vi "main.vi"() -> ()   [LabVIEW 2018]
uses:
  <instrlib>/Tektronix AWG 5000 7000 Series/Public/Configure/Channel/Assign Output Waveform (From Waveform List).vi
  <instrlib>/Tektronix AWG 5000 7000 Series/Tektronix AWG 5000 7000 Series.lvlib
panel:
  in  "Wipe Names on execute":bool
  in  "Name 2":string
  in  "Amp 2":dbl
  in  "Amp 1":dbl
  in  "VISA name":refnum<visa-resource-name>
  in  "Frequency":dbl
  in  "Cant. Freq":dbl
  in  "Name":string
  in  "Max sample rate":dbl
  in  "Amplitude":dbl
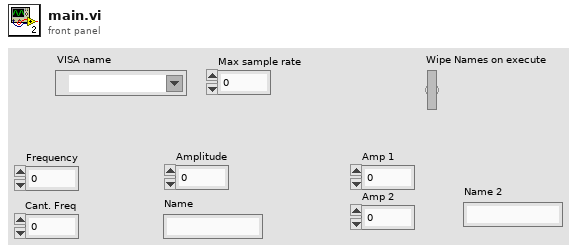
[diagram p1: front panel]
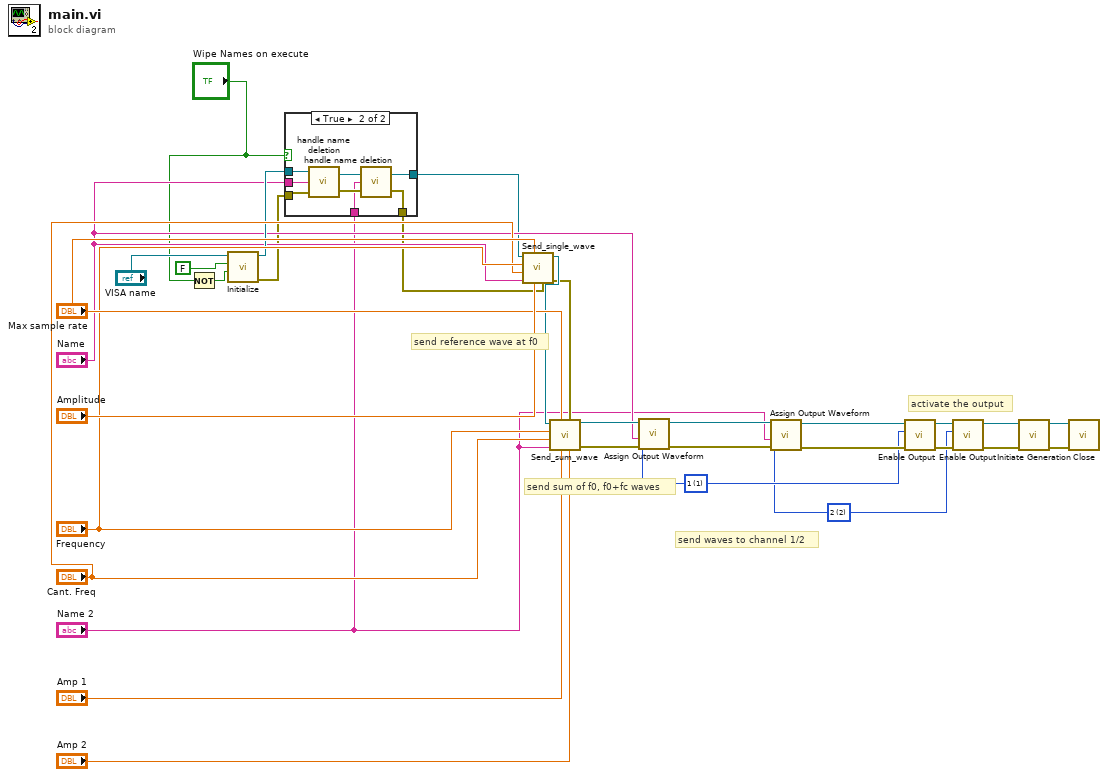
[diagram p0: block diagram]
diagram:
  w16 = u16 1 items=["1"=1, "2"=2, "3"=3, "4"=4] ("Channel Name (1)")
  w13 = u16 2 items=["1"=1, "2"=2, "3"=3, "4"=4] ("Channel Name (1)")
  # "activate the output"
  # "send waves to channel 1/2"
  # "send sum of f0, f0+fc waves"
  # "send reference wave at f0"
  n1 = Not(x="Wipe Names on execute") -> (.not. x?=w3:bool)
  n2 = call <instrlib>:"Initialize.vi"("Reset (False)"=w3, "ID Query (True)"=FALSE, "VISA resource name"="VISA name") -> ("error out"=w6:errorcluster, "VISA resource name out"=w8:refnum<visa-resource-name>)  [unwired: 7 in]
  n3 = case shown="True" "Wipe Names on execute" {
    tunnel: w8 -> [w33 w42]
    tunnel: "Name" -> [_ w41]
    tunnel: w6 -> [w34 w40]
    tunnel: [w33 w39] -> w5
    tunnel: [w34 w38] -> w4
    tunnel: "Name 2" -> [_ w35]
    frame False {
    }
    frame True {
      n4 = call "handle name deletion.vi"("error in (no error)"=w40, "String"=w41, "VISA resource name"=w42) -> ("error out"=w36:errorcluster, "VISA resource name out"=w37:refnum<visa-resource-name>)
      n5 = call "handle name deletion.vi"("error in (no error)"=w36, "String"=w35, "VISA resource name"=w37) -> ("error out"=w38:errorcluster, "VISA resource name out"=w39:refnum<visa-resource-name>)
    }
  }
  n6 = call "Send_single_wave.vi"("error in (no error)"=w4, "Amplitude"="Amplitude", "Max sample rate"="Max sample rate", "Name"="Name", "Cant. Freq"="Cant. Freq", "Frequency"="Frequency", "VISA resource name"=w5) -> ("error out"=w25:errorcluster, "VISA resource name out"=w26:refnum<visa-resource-name>)  [unwired: 3 in]
  n7 = call "Send_sum_wave.vi"("Amp 2"="Amp 2", "error in (no error)"=w25, "Amp 1"="Amp 1", "Max sample rate"="Max sample rate", "Name"="Name 2", "Cant. Freq"="Cant. Freq", "Frequency"="Frequency", "VISA resource name"=w26) -> ("error out"=w21:errorcluster, "VISA resource name out"=w22:refnum<visa-resource-name>)  [unwired: 2 in]
  n8 = call-poly <instrlib>:"Assign Output Waveform.vi"("error in (no error)"=w21, "Waveform"="Name", "Channel Name (1)"=w16, "VISA resource name"=w22) -> ("error out"=w19:errorcluster, "VISA resource name out"=w20:refnum<visa-resource-name>)  [unwired: 6 in]
  n9 = call-poly <instrlib>:"Assign Output Waveform.vi"("error in (no error)"=w19, "Waveform"="Name 2", "Channel Name (1)"=w13, "VISA resource name"=w20) -> ("error out"=w17:errorcluster, "VISA resource name out"=w18:refnum<visa-resource-name>)  [unwired: 6 in]
  n10 = call <instrlib>:"Enable Output.vi"("error in (no error)"=w17, "Channel Name (1)"=w16, "VISA resource name"=w18) -> ("error out"=w14:errorcluster, "VISA resource name out"=w15:refnum<visa-resource-name>)  [unwired: 7 in]
  n11 = call <instrlib>:"Enable Output.vi"("error in (no error)"=w14, "Channel Name (1)"=w13, "VISA resource name"=w15) -> ("error out"=w11:errorcluster, "VISA resource name out"=w12:refnum<visa-resource-name>)  [unwired: 7 in]
  n12 = call <instrlib>:"Initiate Generation.vi"("error in (no error)"=w11, "VISA resource name"=w12) -> ("error out"=w9:errorcluster, "VISA resource name out"=w10:refnum<visa-resource-name>)  [unwired: 8 in]
  n13 = call <instrlib>:"Close.vi"("error in (no error)"=w9, "VISA resource name"=w10) -> ()  [unwired: 9 in, 1 out]
